vi "cno_adjust OB for C.vi"(4 "YY":dbl[](array[numeric]), 5 "constraint weight":dbl, 6 "B":dbl[](array[numeric]), 7 "P":dbl[](array[numeric]), 8 "error in (no error)":errorcluster, 9 "A":dbl[][](array[numeric]), 10 "NC":i32, 11 "OB":dbl[](array[numeric])) -> (0 "error out":errorcluster, 2 "J":dbl, 3 "OB":dbl[](array[numeric]))   [LabVIEW 2014, in "NI_Gmath.lvlib"]
uses:
  NI_Gmath.lvlib
  A x Vector.vi
  Real Matrix Norm.vi
  Real Dot Product.vi
  NI_AALBase.lvlib
  NI_AALPro.lvlib
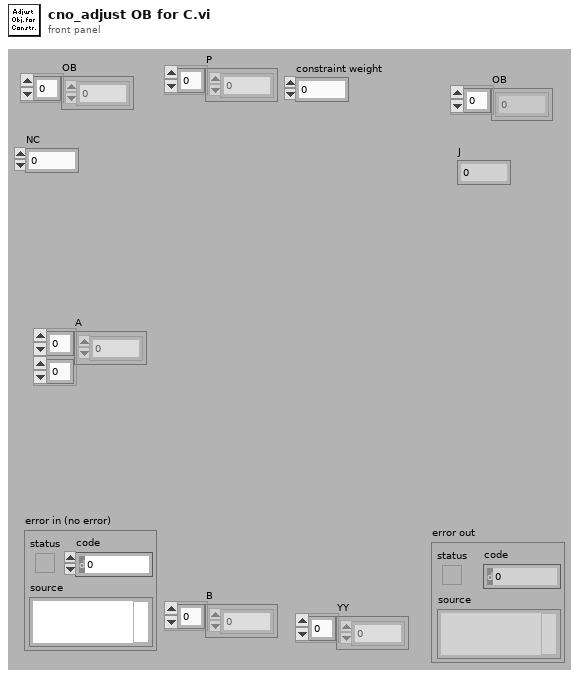
[diagram p1: front panel]
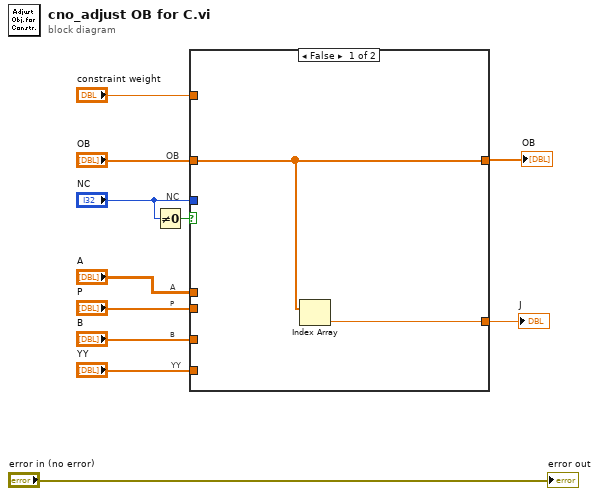
[diagram p0: block diagram]
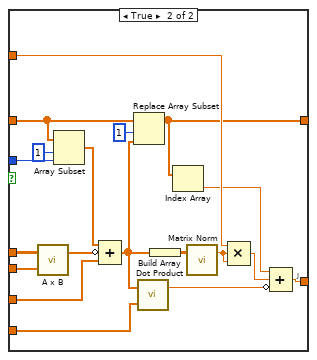
[diagram p2: hidden frame]
diagram:
  # "YY"
  # "P"
  # "B"
  # "A"
  # "NC"
  # "OB"
  n1 = Not Equal To 0?(x="NC") -> (x != 0?=w2:bool)
  n2 = case shown="False" w2 {
    tunnel: "NC" -> [_ w25]
    tunnel: "OB" -> [w13 w26]
    tunnel: "B" -> [_ w28]
    tunnel: "A" -> [_ w31]
    tunnel: "P" -> [_ w30]
    tunnel: "YY" -> [_ w24]
    tunnel: "constraint weight" -> [_ w20]
    tunnel: [w12 w16] -> w6
    tunnel: [w13 w15] -> w9
    frame False {
      n3 = Index Array(array=w13) -> (element=w12:dbl)  [unwired: 1 in]
    }
    frame True {
      # "J"
      n4 = call-poly "A x B.vi"("Vector"=w30, "A"=w31) -> ("A x Vector"=w29:dbl[])  [unwired: 1 out]
      n5 = Array Subset(array=w26, index=1, length=w25) -> (w27:dbl[])
      n6 = Compound Arithmetic op=ADD(w27, invert w29, w28) -> (w23:dbl[])
      n7 = Replace Array Subset(array=w26, new element=w23, index=1) -> (w15:dbl[])
      n8 = call-poly "Dot Product.vi"("Y Vector"=w24, "X Vector"=w23) -> ("X * Y"=w17:dbl)  [unwired: 1 out]
      n9 = Build Array(w23) -> (w22:dbl[][])
      n10 = Index Array(array=w15) -> (element=w19:dbl)  [unwired: 1 in]
      n11 = call-poly "Matrix Norm.vi"("Input Matrix"=w22) -> ("norm"=w21:dbl)  [unwired: 1 in, 1 out]
      n12 = Compound Arithmetic op=MULTIPLY(w20, w21, w21) -> (w18:dbl)
      n13 = Compound Arithmetic op=ADD(w19, w18, invert w17) -> (w16:dbl)
    }
  }
  "OB" <- w9
  "J" <- w6
  "error out" <- "error in (no error)"
